vi "EvaluateAlarms.vi"(8 "error in (no error)":errorcluster, 10 "data":T1, 11 "config in":T5) -> (0 "error out":errorcluster, 3 "config out":T5)   [LabVIEW 2017, in "TrendAlarm.lvlib"]
uses:
  <vilib>/addons/InsightCM/Devices/Shared/Common/TrendAlarm/TrendAlarm.lvlib
  <vilib>/addons/InsightCM/Devices/Shared/Common/TrendAlarm/controls/config.ctl
  <vilib>/addons/InsightCM/Devices/Shared/Common/DataFlow/controls/Data.ctl
  <vilib>/addons/InsightCM/Utilities/DataAccessors/controls/wfmSGL_DVR.ctl
  <vilib>/addons/PointValueMap/controls/PointMap.ctl
  <vilib>/addons/InsightCM/Devices/Shared/Common/DataFlow/controls/Type.ctl
  <vilib>/addons/InsightCM/MessageBus/Base/controls/TrendAlarmRule.ctl
  <vilib>/addons/InsightCM/MessageBus/Base/controls/TrendAlarmLevel.ctl
  <vilib>/addons/InsightCM/MessageBus/Base/controls/AlarmAction.ctl
  <vilib>/addons/InsightCM/MessageBus/Base/controls/KeyValuePair.ctl
  <vilib>/addons/InsightCM/Devices/Shared/Common/TrendAlarm/controls/TransitionCache.ctl
  <vilib>/addons/InsightCM/MessageBus/Base/controls/TrendAlarmTransition.ctl
  <vilib>/addons/PointValueMap/PointValueMap.lvlib
  <vilib>/addons/InsightCM/Devices/Shared/Common/DataFlow/DataFlow.lvlib
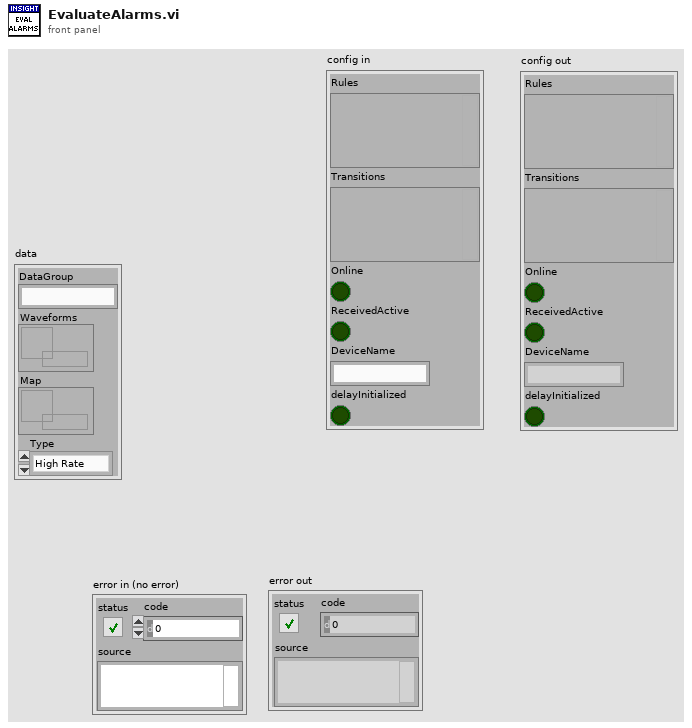
[diagram p1: front panel]
types:
  T1 = typedef "DataFlow.lvlib/Data.ctl" = cluster{"DataGroup":string, "Waveforms":T2, "Map":T3, "Type":T4}
  T2 = typedef "wfmSGL_DVR.ctl" = refnum<data-value>
  T3 = typedef "PointValueMap.lvlib/PointMap.ctl" = refnum<data-value>
  T4 = typedef "DataFlow.lvlib/Type.ctl" = enum16{"High Rate", "Low Rate", "Burst Mode"}
  T5 = typedef "TrendAlarm.lvlib/config.ctl" = cluster{"Rules":variant, "Transitions":variant, "Online":bool, "ReceivedActive":bool, "DeviceName":string, "delayInitialized":bool}
  T6 = typedef "TrendAlarm.lvlib/TransitionCache.ctl" = cluster{"RuleId":string, "MaxSeverity":i32, "LastTransition":T7, "OnTime":timestamp, "OffTime":timestamp}
  T7 = typedef "TrendAlarmTransition.ctl" = cluster{"At":i64, "Severity":i32, "Value":dbl}
  T8 = typedef "TrendAlarmRule.ctl" = cluster{"Id":string, "AssetNodeId":string, "TrendId":string, "Disabled":bool, "OperatingState":string, "Operator":string, "Hysteresis":dbl, "OnDelaySeconds":dbl, "OffDelaySeconds":dbl, "Levels":T9[], "Properties":T11[]}
  T9 = typedef "TrendAlarmLevel.ctl" = cluster{"Severity":i32, "CompareTo":dbl, "Actions":T10[]}
  T10 = typedef "AlarmAction.ctl" = cluster{"Type":string, "Props":T11[]}
  T11 = typedef "KeyValuePair.ctl" = cluster{"Key":string, "Value":string}
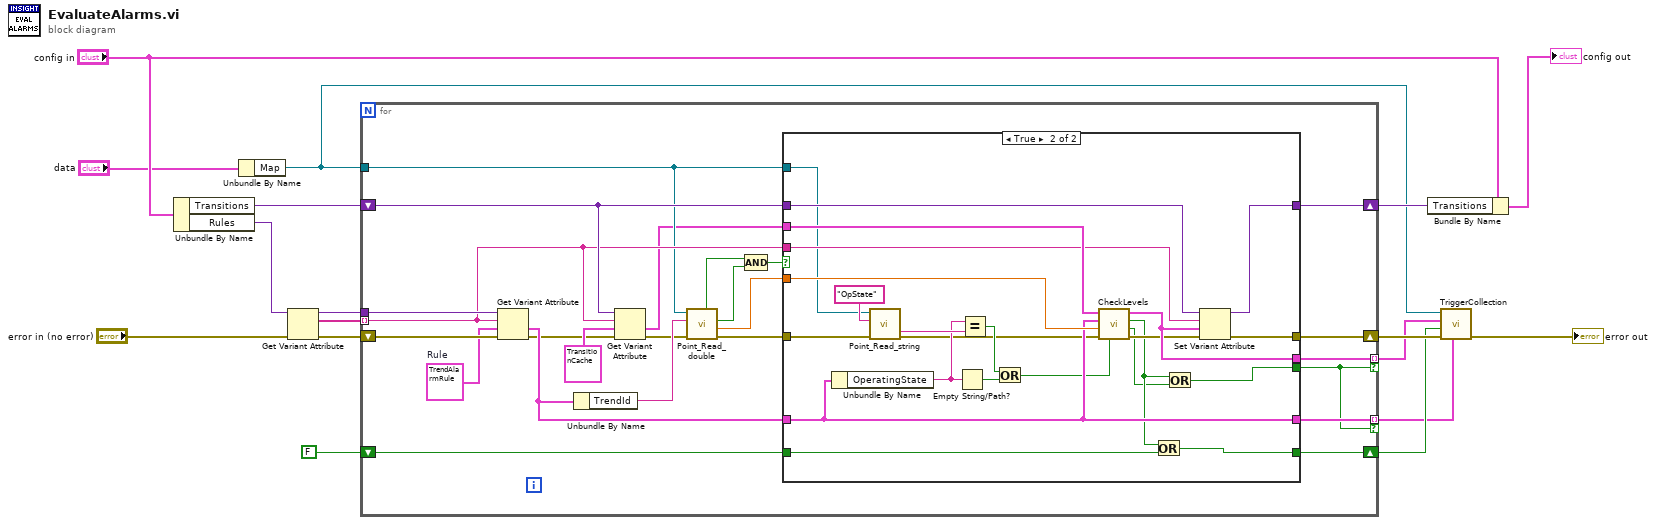
[diagram p0: block diagram]
diagram:
  n1 = Unbundle By Name("config in") -> ("Transitions"=w15:variant, "Rules"=w11:variant)
  n2 = Unbundle By Name("data") -> ("Map"=w2:T3)
  n3 = Get Variant Attribute(Variant=w11, error in="error in (no error)") -> (duplicate Variant=w10:variant, names=w9:string[], error out=w12:errorcluster)  [unwired: 2 in, 1 out]
  n4 = for {
    shift-right: [w36] -> w14
    shift-left: w15 -> [w37]
    shift-right: [w34] -> w6
    shift-left: w12 -> [w41]
    tunnel: w10 -> [w39]
    tunnel: w9 -> [w35] mode=indexing
    tunnel: w2 -> [w27]
    shift-right: [w33] -> w3
    shift-left: FALSE -> [w32]
    tunnel: [w31] -> w4 mode=indexing if=w29
    tunnel: [w30] -> w1 mode=indexing if=w29
    w40 = T8 {"Id"="", "AssetNodeId"="", "TrendId"="", "Disabled"=FALSE, "OperatingState"="", "Operator"="", "Hysteresis"=0.0, "OnDelaySeconds"=0.0, "OffDelaySeconds"=0.0, "Levels"=[], "Properties"=[]}  # Rule
    n5 = Get Variant Attribute(Variant=w39, name=w35, default value (empty Variant)=w40, error in=w41) -> (value=w28:T8, error out=w18:errorcluster)  [unwired: 2 out]
    n6 = Unbundle By Name(w28) -> ("TrendId"=w38:string)
    n7 = Get Variant Attribute(Variant=w37, name=w35, default value (empty Variant)=T6 {"RuleId"="", "MaxSeverity"=0, "LastTransition"={"At"=0, "Severity"=0, "Value"=0.0}, "OnTime"=timestamp(0 s since 1904-01-01), "OffTime"=timestamp(0 s since 1904-01-01)} ("TransitionCache"), error in=w18) -> (value=w19:T6, error out=w25:errorcluster)  [unwired: 2 out]
    n8 = call <vilib>:"Point_Read_double.vi"("Error In"=w25, "Tag"=w38, "Map"=w27) -> ("Error Out"=w20:errorcluster, "Value"=w21:dbl, "Found?"=w23:bool, "Valid?"=w24:bool)  [unwired: 3 in, 2 out]
    n9 = Compound Arithmetic op=AND(w24, w23) -> (w22:bool)
    n10 = case shown="True" w22 {
      tunnel: w21 -> [_ w67]
      tunnel: w20 -> [w43 w51]
      tunnel: w19 -> [_ w66]
      tunnel: w28 -> [_ w50]
      tunnel: w37 -> [w44 w65]
      tunnel: [w44 w64] -> w36
      tunnel: w35 -> [_ w63]
      tunnel: [w43 w62] -> w34
      tunnel: [w42 w61] -> w33
      tunnel: w32 -> [w42 w60]
      tunnel: [_ w59] -> w31
      tunnel: [_ w58] -> w29
      tunnel: [_ w50] -> w30
      tunnel: w27 -> [_ w52]
      frame False {
      }
      frame True {
        n11 = Unbundle By Name(w50) -> ("OperatingState"=w53:string)
        n12 = call <vilib>:"Point_Read_string.vi"("Error In"=w51, "Tag"="OpState", "Map"=w52) -> ("Error Out"=w49:errorcluster, "Value"=w56:string)  [unwired: 3 in, 4 out]
        n13 = Empty String/Path?(string/path=w53) -> (empty?=w54:bool)
        n14 = Equal?(x=w53, y=w56) -> (x = y?=w55:bool)
        n15 = Or(x=w55, y=w54) -> (x .or. y?=w45:bool)
        n16 = call <vilib>:"CheckLevels.vi"("op states match"=w45, "error in (no error)"=w49, "value"=w67, "rule"=w50, "cache in"=w66) -> ("error out"=w48:errorcluster, "update trend"=w46:bool, "update file"=w47:bool, "cache out"=w59:T6)  [unwired: 3 in]
        n17 = Or(x=w47, y=w60) -> (x .or. y?=w61:bool)
        n18 = Or(x=w47, y=w46) -> (x .or. y?=w58:bool)
        n19 = Set Variant Attribute(Variant=w65, name=w63, value=w59, error in=w48) -> (Variant out=w64:variant, error out=w62:errorcluster)  [unwired: 1 out]
      }
    }
  }
  n20 = Bundle By Name(cluster="config in", "Transitions"=w14) -> (→"config out":T5)
  n21 = call <vilib>:"TriggerCollection.vi"("rules"=w1, "error in (no error)"=w6, "collect file"=w3, "updates"=w4, "map"=w2) -> ("error out"=→"error out":errorcluster)  [unwired: 6 in]
